vi "User Event Stop FGV.vi"(8 "error in (no error)":errorcluster, 11 "Action (Get)":T1) -> (0 "error out":errorcluster, 3 "User Event Stop":refnum<user-event>)   [LabVIEW 2018]
doc: "This FGV creates, destroys, and holds the reference to the user event Stop. This event is used to stop all top level VI's.\n\nDefault action is \"Get\", which outputs the user event ref."
uses:
  User Event Stop FGV Action.ctl
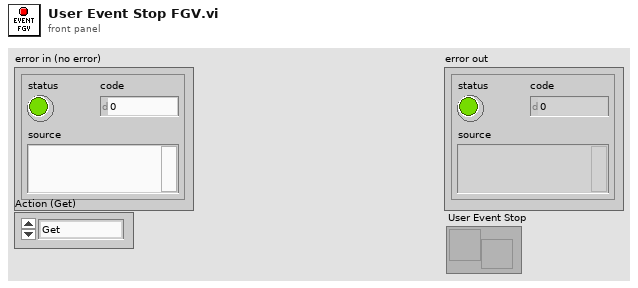
[diagram p1: front panel]
types:
  T1 = typedef "User Event Stop FGV Action.ctl" = enum16{"Get", "Create", "Destroy"}
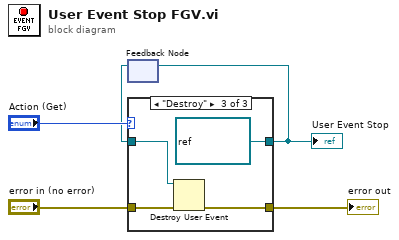
[diagram p0: block diagram]
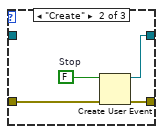
[diagram p3: hidden frame]
diagram:
  n1 = feedback #1() -> (w1:refnum<user-event>)  [unwired: 1 in]
  n2 = case shown="\"Destroy\"" "Action (Get)" {
    tunnel: "error in (no error)" -> [w6 w10 w14]
    tunnel: [w6 w9 w13] -> w3
    tunnel: w1 -> [w7 _ w15]
    tunnel: [w7 w8 refnum<user-event> refnum ("Stop")] -> w2
    frame "Get", Default {
    }
    frame "Create" {
      w11 = FALSE  # Stop
      n3 = Create User Event(user event datatype=w11, error in=w10) -> (user event=w8:refnum<user-event>, error out=w9:errorcluster)
    }
    frame "Destroy" {
      n4 = Destroy User Event(user event=w15, error in=w14) -> (error out=w13:errorcluster)
    }
  }
  "error out" <- w3
  "User Event Stop" <- w2
  n5 = feedback-in #1(w2) -> ()
